vi "Read Prompt SubPanel Ref.vi"(8 "error in (no error)":errorcluster, 11 "Abstract Sensor in":refnum<class "Abstract Sensor.lvclass">) -> (0 "error out":errorcluster, 2 "Prompt SubPanel Ref":refnum<vi>, 3 "Abstract Sensor out":refnum<class "Abstract Sensor.lvclass">)   [LabVIEW 2014]
uses:
  Abstract Sensor.lvclass
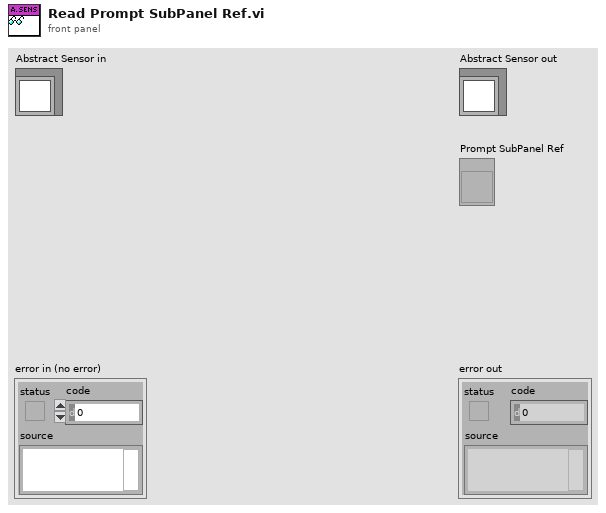
[diagram p1: front panel]
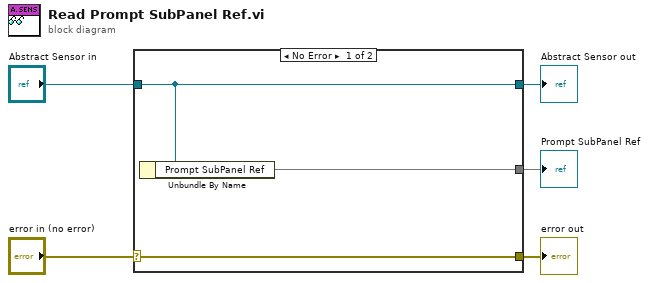
[diagram p0: block diagram]
diagram:
  n1 = case shown="No Error" "error in (no error)" {
    selector: "error in (no error)" -> [w8 w9]
    tunnel: [w8 w9] -> w4
    tunnel: [w7 w10] -> w2
    tunnel: "Abstract Sensor in" -> [w7 w10]
    tunnel: [w6 _] -> w1
    frame No Error {
      n2 = Unbundle By Name(w7) -> ("Prompt SubPanel Ref"=w6)
    }
    frame Error {
    }
  }
  "error out" <- w4
  "Abstract Sensor out" <- w2
  "Prompt SubPanel Ref" <- w1
